vi "Test TCRS Restarting Heating.vi"(8 "error in (no error)":errorcluster, 11 "Thermal Chamber Response Simlator Test In":refnum<class "Thermal Chamber Response Simlator Test.lvclass">) -> (0 "error out":errorcluster, 3 "Thermal Chamber Response Simlator Test Out":refnum<class "Thermal Chamber Response Simlator Test.lvclass">)   [LabVIEW 2020, in "Thermal Chamber Response Simlator Test.lvclass"]
uses:
  Thermal Chamber Response Simlator Test.lvclass
  C:/Program Files (x86)/National Instruments/LabVIEW 2020/vi.lib/Astemes/LUnit/Test Case.lvclass
  Thermal Chamber Response Simlator/Thermal Chamber Response Simlator.lvclass
  Thermal Chamber Response Simlator/Thermal Chamber Response Simlator.lvclass/Thermal Chamber Response Simlator.ctl
  <vilib>/Astemes/LUnit/Test Case.lvclass/Test Case.ctl
  13232ab4-3691-4a04-ae98-dc4ac848fa24.vi
  <vilib>/Astemes/LUnit/Core/LUnit Test Case/Private/Append Pass Result.vi
  <vilib>/Astemes/LUnit/Core/LUnit Test Case/Private/Append Fail Result.vi
  13232ab4-3691-4a04-ae98-dc4ac848fa24.vi/9c5d11cd-9439-4240-a1ee-d9baace9c924.vi
  <vilib>/Astemes/LUnit/Core/LUnit Test Case/Private/Run In UI.vi
  <vilib>/Utility/error.llb/Clear Errors.vi
  Thermal Chamber Response Simlator/Private/Get Current Time if Not Set.vi
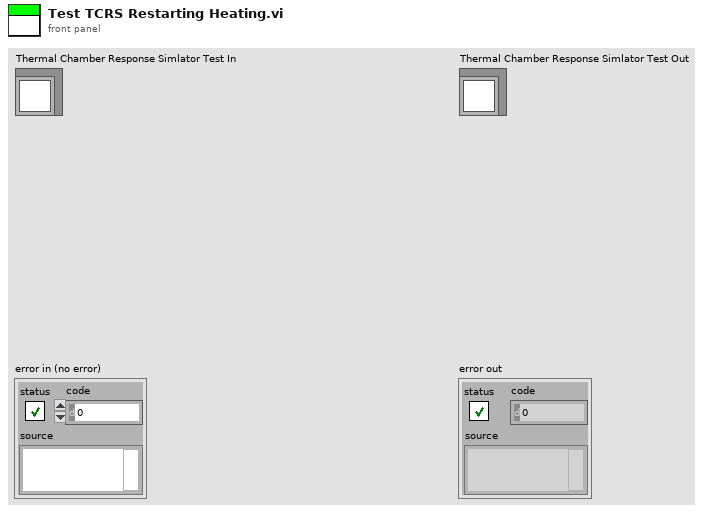
[diagram p1: front panel]
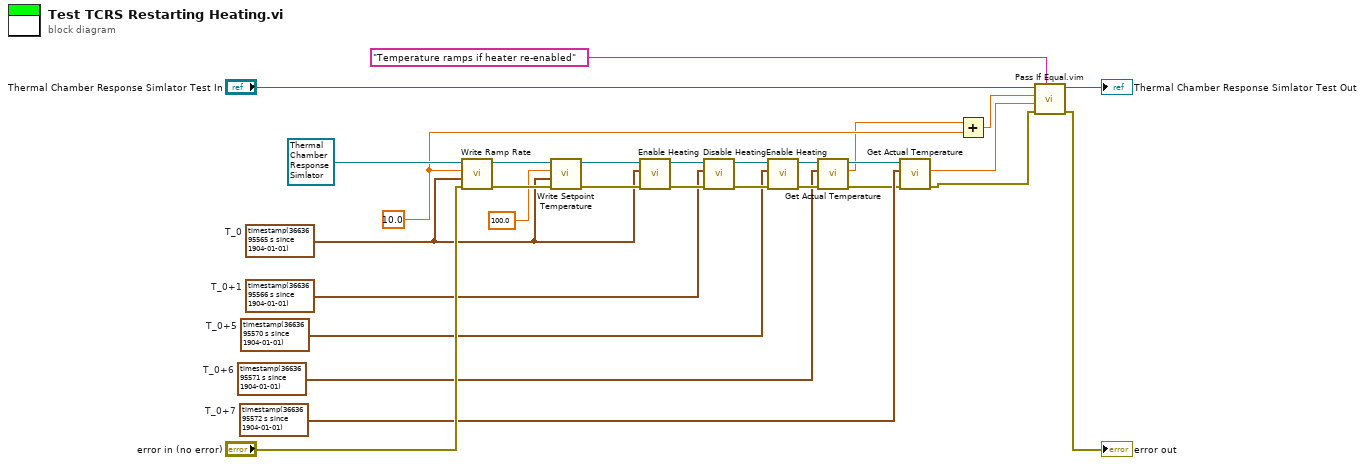
[diagram p0: block diagram]
diagram:
  w7 = timestamp(3663695572 s since 1904-01-01)  # T_0+7
  w13 = timestamp(3663695571 s since 1904-01-01)  # T_0+6
  w16 = timestamp(3663695570 s since 1904-01-01)  # T_0+5
  w17 = timestamp(3663695566 s since 1904-01-01)  # T_0+1
  w14 = 10.0 ("Ramp Rate [degC/s]")
  w1 = timestamp(3663695565 s since 1904-01-01)  # T_0
  n1 = call "Write Ramp Rate.vi"("error in (no error)"="error in (no error)", "Time Stamp"=w1, "Ramp Rate [degC/s]"=w14, "Thermal Chamber Response Simlator In"=refnum<class "Thermal Chamber Response Simlator.lvclass"> refnum ("Thermal Chamber Response Simlator.lvclass")) -> ("error out"=w28:errorcluster, "Thermal Chamber Response Simlator Out"=w11:refnum<class "Thermal Chamber Response Simlator.lvclass">)  [unwired: 6 in]
  n2 = call "Write Setpoint Temperature.vi"("error in (no error)"=w28, "Update Time"=w1, "Setpoint Temperature [degC]"=100.0, "Thermal Chamber Response Simlator In"=w11) -> ("error out"=w12:errorcluster, "Thermal Chamber Response Simlator Out"=w10:refnum<class "Thermal Chamber Response Simlator.lvclass">)  [unwired: 6 in]
  n3 = call "Enable Heating.vi"("error in (no error)"=w12, "Start Time"=w1, "Thermal Chamber Response Simlator In"=w10) -> ("error out"=w22:errorcluster, "Thermal Chamber Response Simlator Out"=w23:refnum<class "Thermal Chamber Response Simlator.lvclass">)  [unwired: 7 in]
  n4 = call "Disable Heating.vi"("error in (no error)"=w22, "Start Time"=w17, "Thermal Chamber Response Simlator In"=w23) -> ("error out"=w21:errorcluster, "Thermal Chamber Response Simlator Out"=w19:refnum<class "Thermal Chamber Response Simlator.lvclass">)  [unwired: 7 in]
  n5 = call "Enable Heating.vi"("error in (no error)"=w21, "Start Time"=w16, "Thermal Chamber Response Simlator In"=w19) -> ("error out"=w20:errorcluster, "Thermal Chamber Response Simlator Out"=w18:refnum<class "Thermal Chamber Response Simlator.lvclass">)  [unwired: 7 in]
  n6 = call "Get Actual Temperature.vi"("error in (no error)"=w20, "Time Stamp"=w13, "Thermal Chamber Response Simlator In"=w18) -> ("error out"=w6:errorcluster, "Actual Temperature [degC]"=w2:dbl, "Thermal Chamber Response Simlator Out"=w8:refnum<class "Thermal Chamber Response Simlator.lvclass">)  [unwired: 6 in]
  n7 = call "Get Actual Temperature.vi"("error in (no error)"=w6, "Time Stamp"=w7, "Thermal Chamber Response Simlator In"=w8) -> ("error out"=w4:errorcluster, "Actual Temperature [degC]"=w5:dbl)  [unwired: 6 in, 1 out]
  n8 = Add(x=w2, y=w14) -> (x+y=w15:dbl)
  n9 = call "Pass If Equal.vim"("Description"="Temperature ramps if heater re-enabled", "error in (no error)"=w4, "Actual"=w5, "Expected"=w15, "LUnit Test Case In"="Thermal Chamber Response Simlator Test In") -> ("error out"=→"error out":errorcluster, "LUnit Test Case Out"=→"Thermal Chamber Response Simlator Test Out":refnum<class "Thermal Chamber Response Simlator Test.lvclass">)  [unwired: 5 in]
